vi "Read Pin Map.vi"(8 "error in (no error)":errorcluster, 11 "NI-DAQ in":refnum<class "NI-DAQ.lvclass">) -> (0 "error out":errorcluster, 2 "Pin Map":T1={"Region Valves"=[49, 52, 0, 0], "Extra Valves"=[[[0.0, 48.0, 0.0, 0.0, 0.0]]], "Tool Primary Valve"=51, "Tool Secondary Valve"=50, "Region Sensors"=[37, 41, 37], "Extra Sensors"=[[[36.0, 37.0, 0.0, 0.0]]], "Tool Primary Sensor"=39.0, "Tool Secondary Sensor"=38.0, "Compression Sensor"=31.0, "5V"=50, "Dispenser Sensor"=0.0, "Light Curtain"=50}, 3 "NI-DAQ out":refnum<class "NI-DAQ.lvclass">)   [LabVIEW 2021, in "NI-DAQ.lvclass"]
uses:
  NI-DAQ.lvclass
  Pin Map.ctl
  <vilib>/Utility/file.llb/Read Delimited Spreadsheet (DBL).vi
  I-O.lvclass
panel:
  out "extra valves":i32[][][](array[numeric])
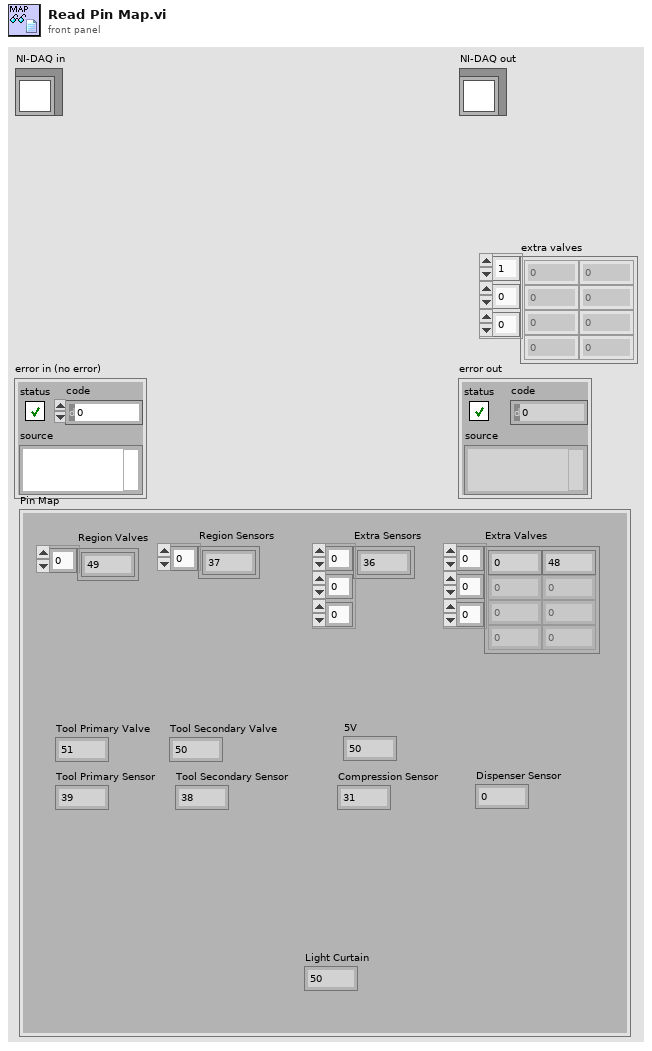
[diagram p1: front panel]
types:
  T1 = typedef "I-O.lvclass/Pin Map.ctl" = cluster{"Region Valves":i32[], "Extra Valves":dbl[][][], "Tool Primary Valve":i32, "Tool Secondary Valve":i32, "Region Sensors":i32[], "Extra Sensors":dbl[][][], "Tool Primary Sensor":dbl, "Tool Secondary Sensor":dbl, "Compression Sensor":dbl, "5V":i32, "Dispenser Sensor":dbl, "Light Curtain":i32}
  T2 = typedef "File Paths.ctl" = cluster{"Glue Pattern Folder":path, "Carrier Tray Folder":path, "Pick Up Tool Fixture Folder":path, "Components Folder":path, "Bellows Tool Offset.txt":path, "Pick Up Tool Offset.txt":path, "Dispense Tip Offset.txt":path, "Log Files":path, "Gantry Assembly Map.txt":path, "Syringe and offset map.txt":path, "Controllers Folder":path, "Local dbase config":path}
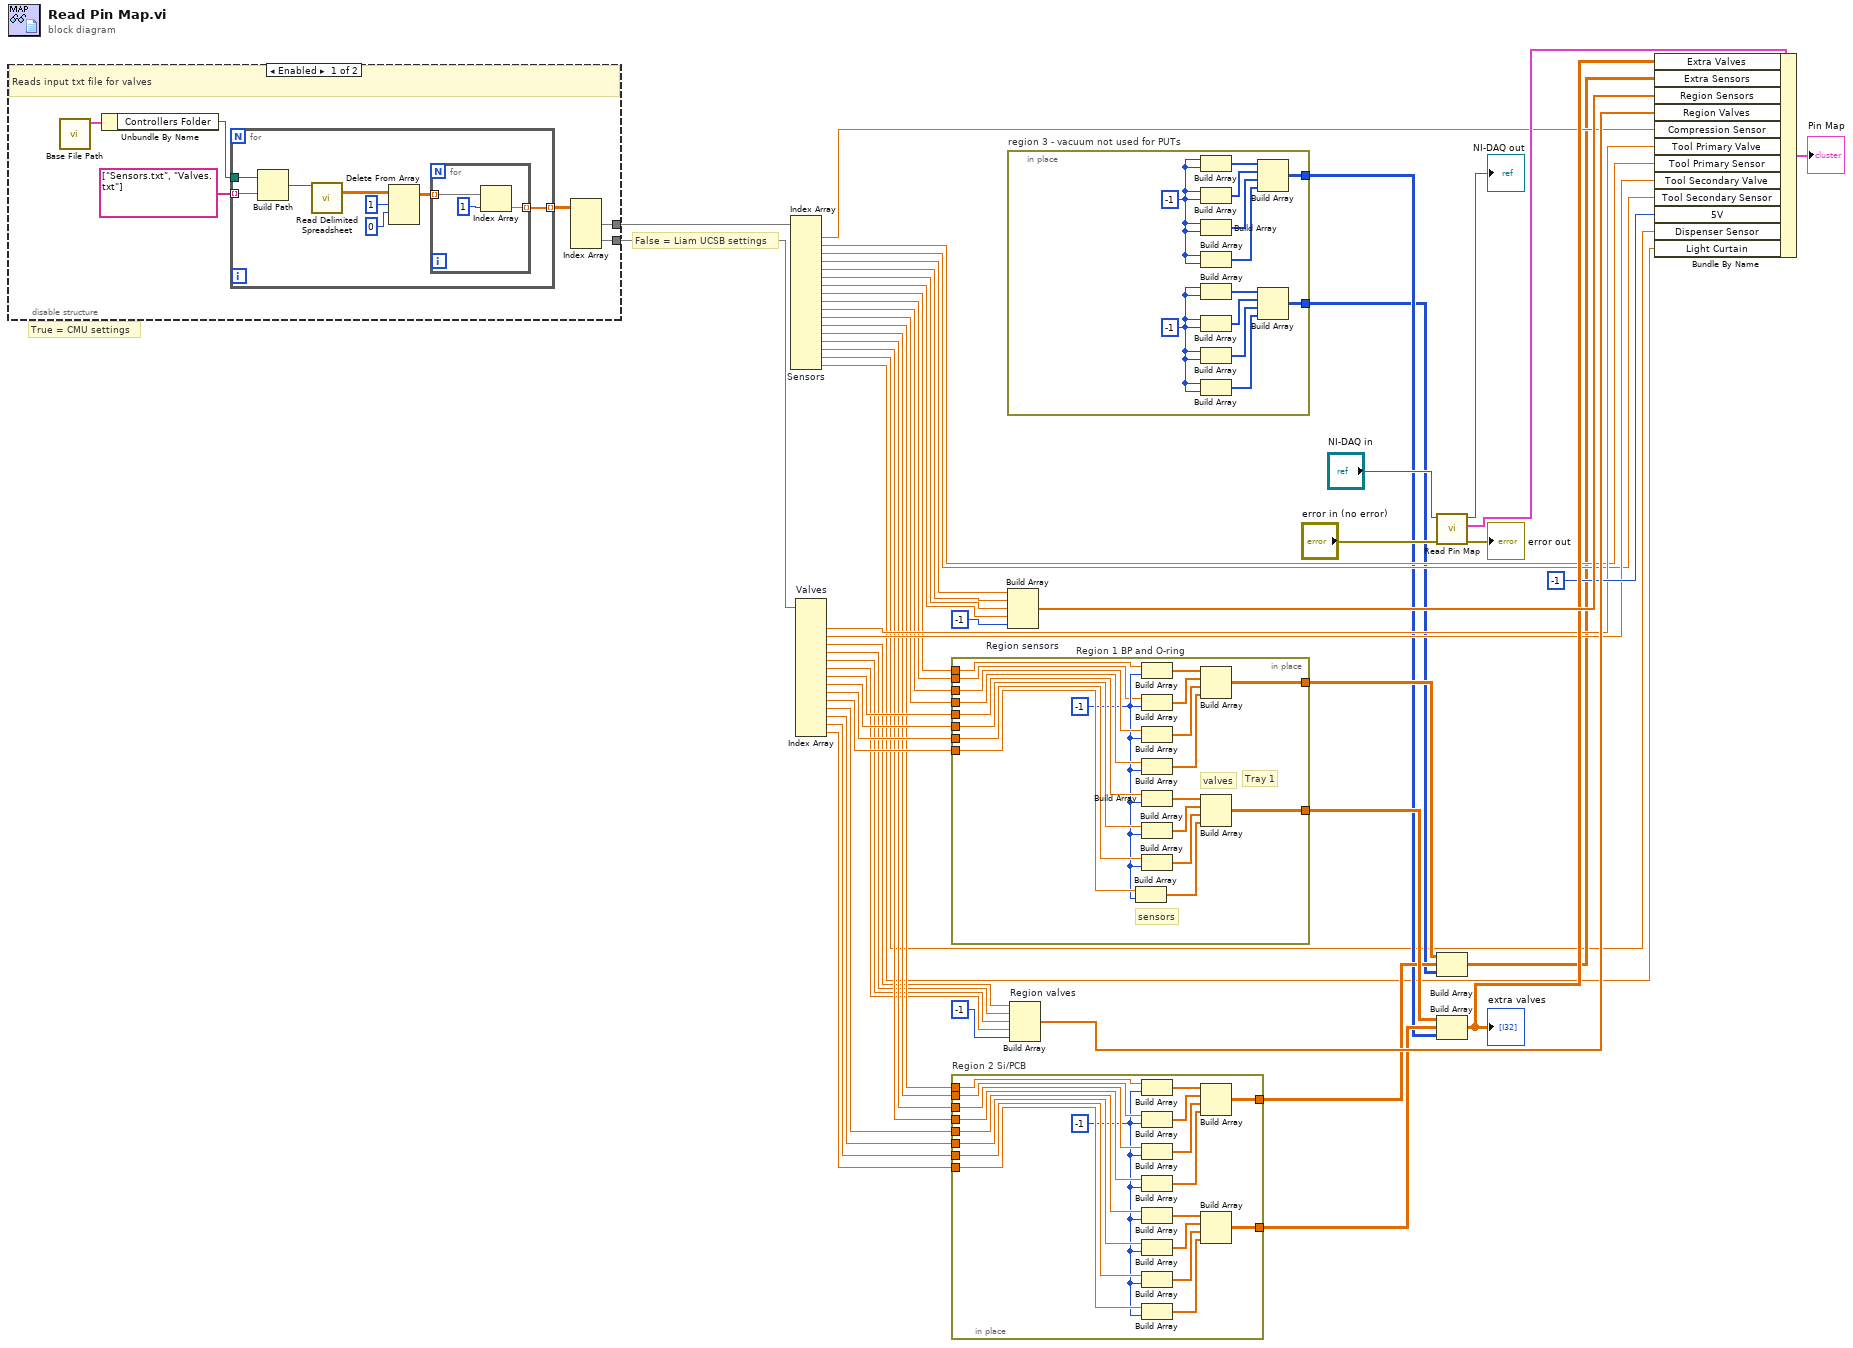
[diagram p0: block diagram]
diagram:
  # "False = Liam UCSB settings"
  # "True = CMU settings"
  n1 = disable-structure shown="Enabled" {
    disable-tunnel: [w54 _] -> w52
    disable-tunnel: [w53 _] -> w51
    frame Enabled {
      # "Reads input txt file for valves"
      n2 = call "Base File Path.vi"() -> ("Paths Out"=w58:T2)  [unwired: 11 in]
      n3 = Unbundle By Name(w58) -> ("Controllers Folder"=w56:path)
      n4 = for {
        tunnel: string[] ["Sensors.txt", "Valves.txt"] -> [w64] mode=indexing
        tunnel: w56 -> [w65]
        tunnel: [w59] -> w55 mode=indexing
        n5 = Build Path(base path=w65, name or relative path=w64) -> (appended path=w66:path)
        n6 = call-poly <vilib>:"Read Delimited Spreadsheet.vi"("file path (dialog if empty)"=w66) -> ("all rows"=w63:dbl[][])  [unwired: 9 in, 5 out]
        n7 = Delete From Array(array=w63, length=1, index (row)=0) -> (array with subset deleted=w60:dbl[][])  [unwired: 1 in, 1 out]
        n8 = for {
          tunnel: w60 -> [w69] mode=indexing
          tunnel: [w68] -> w59 mode=indexing
          n9 = Index Array(array=w69, index=1) -> (element=w68:dbl)
        }
      }
      n10 = Index Array(array=w55) -> (element #1=w54:dbl[], element #2=w53:dbl[])  [unwired: 4 in]
    }
    frame Disabled {
    }
  }
  n11 = Index Array "Sensors"(array=w52) -> (element #1=w38:dbl, element #2=w37:dbl, element #3=w36:dbl, element #4=w17:dbl, element #5=w16:dbl, element #6=w15:dbl, element #7=w14:dbl, element #8=w24:dbl, element #9=w29:dbl, element #10=w23:dbl, element #11=w22:dbl, element #12=w21:dbl, element #13=w18:dbl, element #14=w19:dbl, element #15=w20:dbl, element #16=w2:dbl, element #17=w1:dbl)  [unwired: 17 in]
  n12 = Index Array "Valves"(array=w51) -> (element #2=w40:dbl, element #3=w39:dbl, element #4=w6:dbl, element #5=w5:dbl, element #6=w4:dbl, element #7=w3:dbl, element #8=w35:dbl, element #9=w34:dbl, element #10=w27:dbl, element #11=w33:dbl, element #12=w32:dbl, element #13=w26:dbl, element #14=w31:dbl, element #15=w25:dbl)  [unwired: 15 in, 1 out]
  n13 = in-place "Region 1 BP and O-ring" {
    in-place-border: [w88] -> w12
    in-place-border: [w87] -> w11
    in-place-border: w35 -> [w86]
    in-place-border: w34 -> [w82]
    in-place-border: w33 -> [w80]
    in-place-border: w29 -> [w74]
    in-place-border: w27 -> [w81]
    in-place-border: w24 -> [w75]
    in-place-border: w23 -> [w78]
    in-place-border: w22 -> [w77]
    w76 = -1
    # "sensors"
    # "valves"
    # "Tray 1"
    n14 = Build Array(w80, w76) -> (w72:dbl[])
    n15 = Build Array(w75, w76) -> (w83:dbl[])
    n16 = Build Array(w74, w76) -> (w79:dbl[])
    n17 = Build Array(w78, w76) -> (w71:dbl[])
    n18 = Build Array(w77, w76) -> (w70:dbl[])
    n19 = Build Array(w86, w76) -> (w85:dbl[])
    n20 = Build Array(w82, w76) -> (w84:dbl[])
    n21 = Build Array(w81, w76) -> (w73:dbl[])
    n22 = Build Array(w83, w79, w71, w70) -> (w87:dbl[][])
    n23 = Build Array(w85, w84, w73, w72) -> (w88:dbl[][])
  }
  n24 = in-place "Region 2 Si/PCB" {
    in-place-border: [w107] -> w13
    in-place-border: w32 -> [w104]
    in-place-border: w31 -> [w102]
    in-place-border: w26 -> [w103]
    in-place-border: w25 -> [w101]
    in-place-border: w21 -> [w100]
    in-place-border: w20 -> [w98]
    in-place-border: w19 -> [w97]
    in-place-border: w18 -> [w96]
    in-place-border: [w93] -> w10
    w94 = -1
    n25 = Build Array(w100, w94) -> (w99:dbl[])
    n26 = Build Array(w96, w94) -> (w95:dbl[])
    n27 = Build Array(w97, w94) -> (w90:dbl[])
    n28 = Build Array(w98, w94) -> (w89:dbl[])
    n29 = Build Array(w104, w94) -> (w105:dbl[])
    n30 = Build Array(w103, w94) -> (w106:dbl[])
    n31 = Build Array(w102, w94) -> (w91:dbl[])
    n32 = Build Array(w101, w94) -> (w92:dbl[])
    n33 = Build Array(w99, w95, w90, w89) -> (w93:dbl[][])
    n34 = Build Array(w105, w106, w91, w92) -> (w107:dbl[][])
  }
  n35 = in-place "region 3 - vacuum not used for PUTs" {
    in-place-border: [w119] -> w9
    in-place-border: [w118] -> w8
    w108 = -1
    w109 = -1
    n36 = Build Array(w109, w109) -> (w117:i32[])
    n37 = Build Array(w109, w109) -> (w116:i32[])
    n38 = Build Array(w109, w109) -> (w115:i32[])
    n39 = Build Array(w109, w109) -> (w114:i32[])
    n40 = Build Array(w108, w108) -> (w113:i32[])
    n41 = Build Array(w108, w108) -> (w111:i32[])
    n42 = Build Array(w108, w108) -> (w112:i32[])
    n43 = Build Array(w108, w108) -> (w110:i32[])
    n44 = Build Array(w117, w116, w115, w114) -> (w119:i32[][])
    n45 = Build Array(w113, w111, w112, w110) -> (w118:i32[][])
  }
  n46 = Build Array "Region sensors"(w17, w16, w15, w14, -1) -> (w43:dbl[])
  n47 = Build Array "Region valves"(w6, w5, w4, w3, -1) -> (w44:dbl[])
  n48 = call-parent "Read Pin Map.vi"("error in (no error)"="error in (no error)", "I-O in"="NI-DAQ in") -> ("error out"=→"error out":errorcluster, "Pin Map 2"=w46:T1, "I-O out"=→"NI-DAQ out":refnum<class "NI-DAQ.lvclass">)  [unwired: 7 in]
  n49 = Build Array(w11, w10, w8) -> (w28:dbl[][][])
  n50 = Build Array(w12, w13, w9) -> (w42:dbl[][][])
  "extra valves" <- w42
  n51 = Bundle By Name(cluster=w46, "Extra Valves"=w42, "Extra Sensors"=w28, "Region Sensors"=w43, "Region Valves"=w44, "Compression Sensor"=w38, "Tool Primary Valve"=w40, "Tool Primary Sensor"=w37, "Tool Secondary Valve"=w39, "Tool Secondary Sensor"=w36, "5V"=-1, "Dispenser Sensor"=w2, "Light Curtain"=w1) -> (→"Pin Map":T1)
